vi "SEQ Lossy Queue.vi"(8 "error in":errorcluster, 11 "SEQ Data":T1) -> (0 "error out":errorcluster)   [LabVIEW 2019, in "Image.lvlib"]
uses:
  Image.lvlib
  SEQ Data.ctl
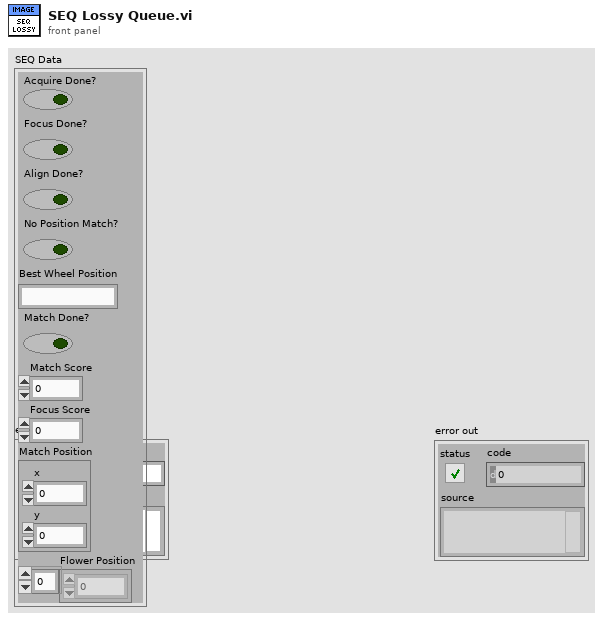
[diagram p1: front panel]
types:
  T1 = typedef "Image.lvlib/SEQ Data.ctl" = cluster{"Acquire Done?":bool, "Focus Done?":bool, "Align Done?":bool, "No Position Match?":bool, "Best Wheel Position":string, "Match Done?":bool, "Match Score":dbl, "Focus Score":dbl, "Match Position":cluster{"x":sgl, "y":sgl}, "Flower Position":i32[]}
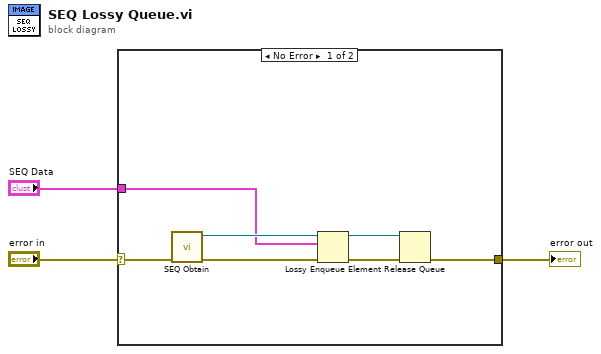
[diagram p0: block diagram]
diagram:
  n1 = case shown="No Error" "error in" {
    selector: "error in" -> [w7 w11]
    tunnel: [w8 w11] -> w2
    tunnel: "SEQ Data" -> [w4 _]
    frame No Error {
      n2 = call "SEQ Obtain.vi"("error in"=w7) -> ("error out"=w6:errorcluster, "queue out"=w5:refnum<queue>)  [unwired: 9 in]
      n3 = Lossy Enqueue Element(queue=w5, element=w4, error in (no error)=w6) -> (queue out=w9:refnum<queue>, error out=w10:errorcluster)  [unwired: 2 out]
      n4 = Release Queue(queue=w9, error in (no error)=w10) -> (error out=w8:errorcluster)  [unwired: 1 in, 2 out]
    }
    frame Error {
    }
  }
  "error out" <- w2
